vi "NewProj.vi"(3 "entrée d'erreur":errorcluster) -> (0 "sortie d'erreur":errorcluster, 2 "NomProjet":string)   [LabVIEW 2017]
panel:
  in  "New project name (3 to 6 characters) :":string
  in  "Creer":bool
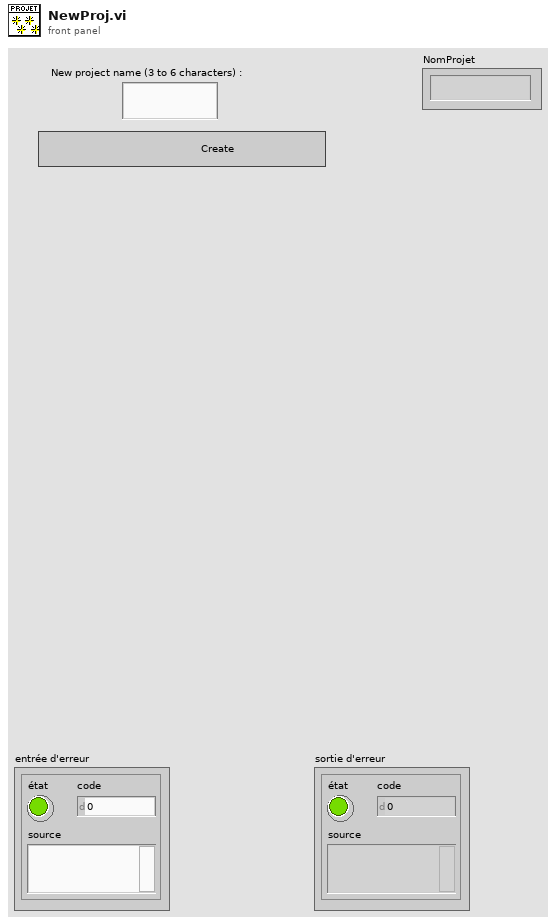
[diagram p1: front panel]
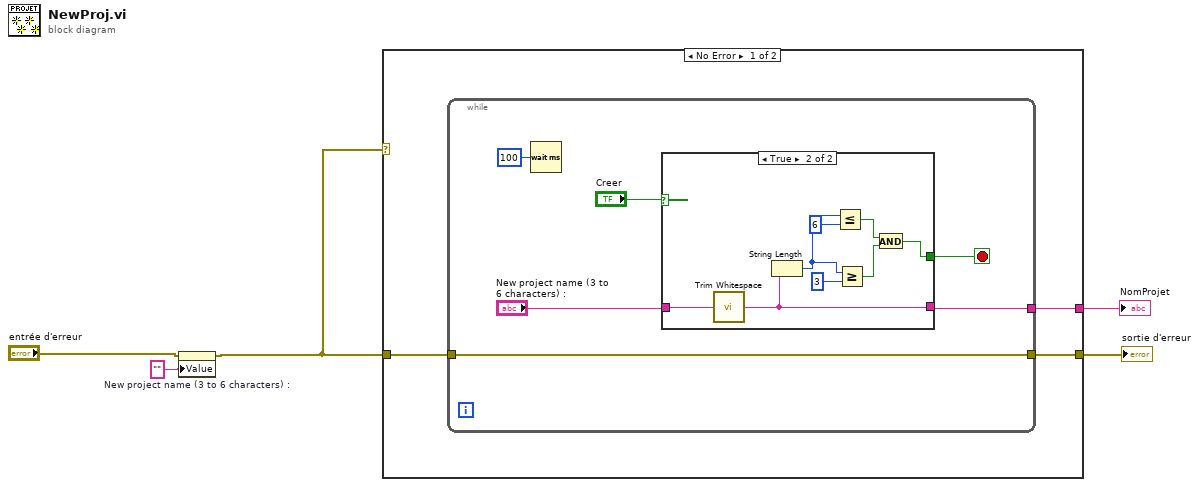
[diagram p0: block diagram]
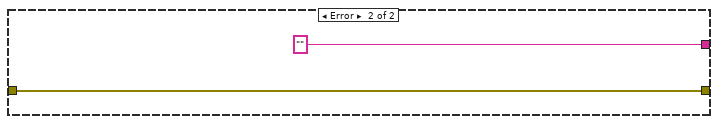
[diagram p3: hidden frame]
diagram:
  n1 = property on="New project name (3 to 6 characters) :" class="Str"(error in="entrée d'erreur", "Value"="" ("New project name :")) -> (error out=w2:errorcluster)  [unwired: 1 in, 1 out]
  n2 = case shown="No Error" w2 {
    tunnel: [w7 w26] -> w5
    tunnel: w2 -> [w6 w26]
    tunnel: [w8 ""] -> w4
    frame No Error {
      n3 = while {
        tunnel: [w10] -> w8
        tunnel: [w13] -> w7
        tunnel: w6 -> [w13]
        stop <- w9 stop-if-true
        n4 = Wait (ms)(milliseconds to wait=u32 100 ("attente (ms)")) -> ()  [unwired: 1 out]
        n5 = case shown="True" "Creer" {
          selector: "Creer" -> [w15 _]
          tunnel: "New project name (3 to 6 characters) :" -> [w16 w23]
          tunnel: [w16 w22] -> w10
          tunnel: [w15 w17] -> w9
          frame False {
          }
          frame True {
            n6 = call <vilib>:"Trim Whitespace.vi"("string"=w23) -> ("trimmed string"=w22:string)  [unwired: 1 in]
            n7 = String Length(string=w22) -> (length=w21:i32)
            n8 = Less Or Equal?(x=w21, y=6) -> (x <= y?=w19:bool)
            n9 = Greater Or Equal?(x=w21, y=3) -> (x >= y?=w18:bool)
            n10 = And(x=w19, y=w18) -> (x .and. y?=w17:bool)
          }
        }
      }
    }
    frame Error {
    }
  }
  "sortie d'erreur" <- w5
  "NomProjet" <- w4
